vi "example-ParamClusterControl.vi"() -> ()   [LabVIEW 2021]
panel:
  in  "Serial port":refnum<visa-resource-name>="COM7"
  in  "Cluster":T1
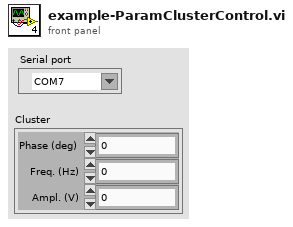
[diagram p1: front panel]
types:
  T1 = cluster{"Phase (deg)":dbl, "Freq. (Hz)":dbl, "Ampl. (V)":dbl}
  T2 = cluster{"Operation":enum16{"read", "write"}, "Data":string, "Queue":refnum<queue>}
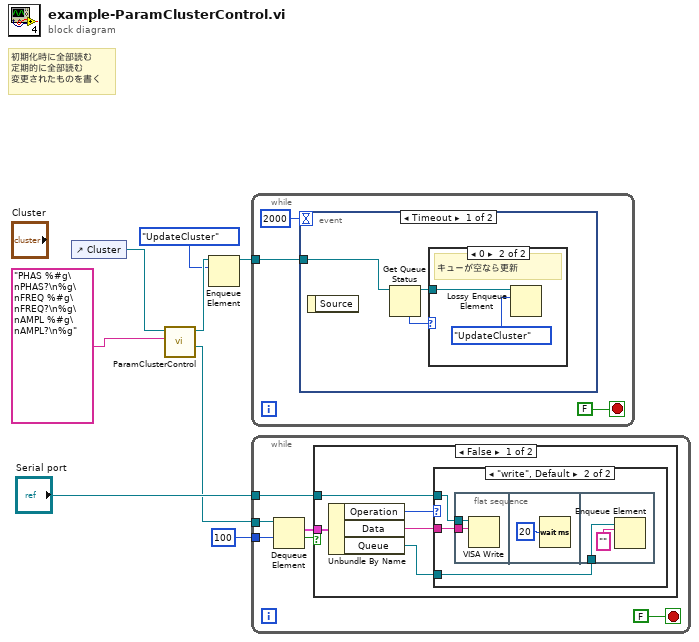
[diagram p0: block diagram]
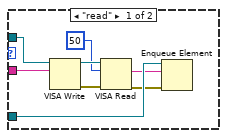
[diagram p2: hidden frame]
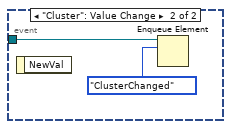
[diagram p5: hidden frame]
diagram:
  # "初期化時に全部読む\n定期的に全部読む\n変更されたものを書く"
  n1 = control-ref of="Cluster"() -> (w8:refnum<vi>)
  n2 = call "ParamClusterControl.vi"("SetGetCommands"="PHAS %#g\nPHAS?\n%g\nFREQ %#g\nFREQ?\n%g\nAMPL %#g\nAMPL?\n%g", "Cluster ref"=w8) -> ("IO queue out"=w1:refnum<queue>, "Command queue"=w5:refnum<queue>)  [unwired: 8 in]
  n3 = Enqueue Element(queue=w5, element=enum16{"UpdateCluster", "ClusterChanged"}."UpdateCluster") -> (queue out=w6:refnum<queue>)  [unwired: 2 in, 2 out]
  n4 = while {
    tunnel: w6 -> [w10]
    stop <- FALSE stop-if-true
    n5 = event shown="[0] Timeout" {
      selector: _ -> [_ _]
      dyn-events: _ -> [_ _]
      timeout: 2000 -> [_ _]
      tunnel: w10 -> [w14 w18]
      event Timeout {
        n6 = event-data() -> ()  [unwired: 1 in, 1 out]
        n7 = Get Queue Status(queue=w14) -> (queue out=w12:refnum<queue>, # elements in queue=w13:i32)  [unwired: 2 in, 6 out]
        n8 = case shown="0" w13 {
          tunnel: w12 -> [_ w16]
          frame Default {
          }
          frame 0 {
            # "キューが空なら更新"
            n9 = Lossy Enqueue Element(queue=w16, element=enum16{"UpdateCluster", "ClusterChanged"}."UpdateCluster") -> ()  [unwired: 1 in, 4 out]
          }
        }
      }
      event "Cluster": Value Change {
        n10 = event-data() -> ()  [unwired: 1 in, 1 out]
        n11 = Enqueue Element(queue=w18, element=enum16{"UpdateCluster", "ClusterChanged"}."ClusterChanged") -> ()  [unwired: 2 in, 3 out]
      }
    }
  }
  n12 = while {
    tunnel: w1 -> [w24]
    tunnel: "Serial port" -> [w20]
    tunnel: 100 ("timeout in ms (-1)") -> [w19]
    stop <- FALSE stop-if-true
    n13 = Dequeue Element(queue=w24, timeout in ms (-1)=w19) -> (element=w23:T2, timed out?=w22:bool)  [unwired: 1 in, 2 out]
    n14 = case shown="False" w22 {
      tunnel: w23 -> [w29 _]
      tunnel: w20 -> [w27 _]
      frame False {
        n15 = Unbundle By Name(w29) -> ("Operation"=w26:enum16{"read", "write"}, "Data"=w25:string, "Queue"=w28:refnum<queue>)
        n16 = case shown="\"write\", Default" w26 {
          tunnel: w25 -> [w36 w38]
          tunnel: w28 -> [w33 w40]
          tunnel: w27 -> [w37 w39]
          frame "read" {
            n17 = VISA Write(VISA resource name=w37, write buffer=w36) -> (VISA resource name out=w34:refnum<visa-resource-name>, error out=w35:errorcluster)  [unwired: 1 in, 1 out]
            n18 = VISA Read(VISA resource name=w34, byte count=u32 50, error in (no error)=w35) -> (read buffer=w32:string, error out=w31:errorcluster)  [unwired: 2 out]
            n19 = Enqueue Element(queue=w33, element=w32, error in (no error)=w31) -> ()  [unwired: 1 in, 3 out]
          }
          frame "write", Default {
            n20 = flat-sequence {
              tunnel: w39 -> [w42]
              tunnel: w38 -> [w41]
              tunnel: w40 -> [w45]
              frame #0 {
                n21 = VISA Write(VISA resource name=w42, write buffer=w41) -> ()  [unwired: 1 in, 3 out]
              }
              frame #1 {
                n22 = Wait (ms)(milliseconds to wait=u32 20) -> ()  [unwired: 1 out]
              }
              frame #2 {
                n23 = Enqueue Element(queue=w45, element="") -> ()  [unwired: 2 in, 3 out]
              }
            }
          }
        }
      }
      frame True {
      }
    }
  }
